vi "saveImage.vi"(8 "错误输入（无错误） 2":errorcluster caption="错误输入（无错误）", 10 "输入文件名":string, 11 "VISA资源名称":refnum<visa-resource-name>) -> (0 "错误输出":errorcluster, 3 "VISA资源名称输出":refnum<visa-resource-name>)   [LabVIEW 2014]
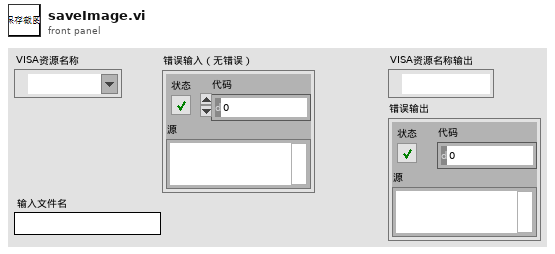
[diagram p1: front panel]
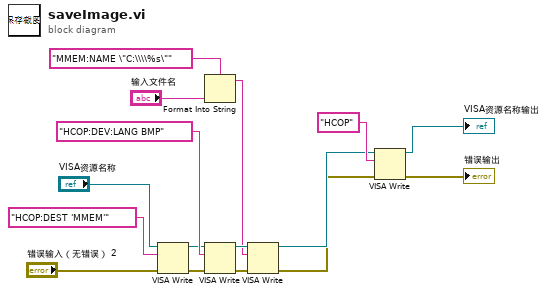
[diagram p0: block diagram]
diagram:
  n1 = VISA Write(VISA resource name="VISA资源名称", write buffer="HCOP:DEST 'MMEM'" ("写入缓冲区"), error in (no error)="错误输入（无错误） 2") -> (VISA resource name out=w9:refnum<visa-resource-name>, error out=w8:errorcluster)  [unwired: 1 out]
  n2 = Format Into String(format string="MMEM:NAME \"C:\\\\%s\"" ("格式字符串"), "输入文件名") -> (resulting string=w12:string)  [unwired: 2 in, 1 out]
  n3 = VISA Write(VISA resource name=w9, write buffer="HCOP:DEV:LANG BMP" ("格式字符串"), error in (no error)=w8) -> (VISA resource name out=w16:refnum<visa-resource-name>, error out=w15:errorcluster)  [unwired: 1 out]
  n4 = VISA Write(VISA resource name=w16, write buffer=w12, error in (no error)=w15) -> (VISA resource name out=w2:refnum<visa-resource-name>, error out=w1:errorcluster)  [unwired: 1 out]
  n5 = VISA Write(VISA resource name=w2, write buffer="HCOP" ("写入缓冲区"), error in (no error)=w1) -> (VISA resource name out=→"VISA资源名称输出":refnum<visa-resource-name>, error out=→"错误输出":errorcluster)  [unwired: 1 out]
